vi "Repeat String.vi"(1 "Num of Repeat":i32=1, 2 "String to Repeat":string) -> (0 "Repeated String":string)   [LabVIEW 2019]
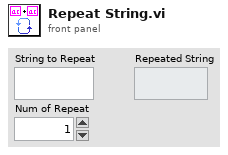
[diagram p1: front panel]
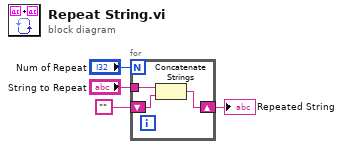
[diagram p0: block diagram]
diagram:
  n1 = for {
    N: "Num of Repeat" -> [_]
    tunnel: "String to Repeat" -> [w7]
    shift-right: [w6] -> w1
    shift-left: "" -> [w5]
    n2 = Concatenate Strings(w7, w5) -> (w6:string)
  }
  "Repeated String" <- w1
